vi "18-1.vi"() -> ()   [LabVIEW 2019, in "18.lvlib"]
uses:
  18.lvlib
panel:
  in  "Sample?":bool
  out "Snailfish Number Sum Magnitude":u64
  in  "Sample Index":i32
  out "Snailfish Number Sum Result":string
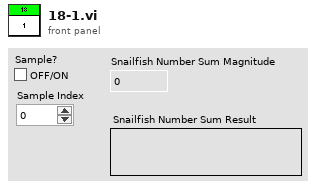
[diagram p1: front panel]
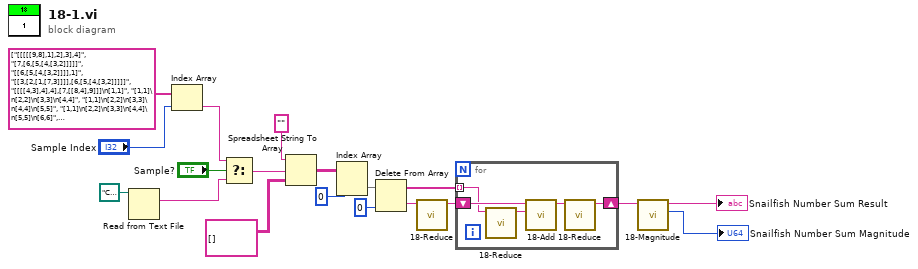
[diagram p0: block diagram]
diagram:
  n1 = Read from Text File(file (use dialog)=path "C:/Users/craig.walker/Documents/GitHub/lv2019-Advent-of-Code-2021/18/input.txt") -> (text=w2:string)  [unwired: 3 in, 3 out]
  n2 = Index Array(array=string[] ["[[[[[9,8],1],2],3],4]", "[7,[6,[5,[4,[3,2]]]]]", "[[6,[5,[4,[3,2]]]],1]", "[[3,[2,[1,[7,3]]]],[6,[5,[4,[3,2]]]]]", "[[[[4,3],4],4],[7,[[8,4],9]]]\n[1,1]", "[1,1]\n[2,2]\n[3,3]\n[4,4]", "[1,1]\n[2,2]\n[3,3]\n[4,4]\n[5,5]", "[1,1]\n[2,2]\n[3,3]\n[4,4]\n[5,5]\n[6,6]", "[[[0,[4,5]],[0,0]],[[[4,5],[2,6]],[9,5]]]\n[7,[[[3,7],[4,3]],[[6,3],[8,8]]]]\n[[2,[[0,8],[3,4]]],[[[6,7],1],[7,[1,6]]]]\n[[[[2,4],7],[6,[0,5]]],[[[6,8],[2,8]],[[2,1],[4,5]]]]\n[7,[5,[[3,8],[1,4]]]]\n[[2,[2,2]],[8,[8,1]]]\n[2,9]\n[1,[[[9,3],9],[[9,0],[0,7]]]]\n[[[5,[7,4]],7],1]\n[[[[4,2],2],6],[8,7]]", "[9,1]", "[[[0,[5,8]],[[1,7],[9,6]]],[[4,[1,2]],[[1,4],2]]]\n[[[5,[2,8]],4],[5,[[9,9],0]]]\n[6,[[[6,2],[5,6]],[[7,6],[4,7]]]]\n[[[6,[0,7]],[0,9]],[4,[9,[9,0]]]]\n[[[7,[6,4]],[3,[1,3]]],[[[5,5],1],9]]\n[[6,[[7,3],[3,2]]],[[[3,8],[5,7]],4]]\n[[[[5,4],[7,7]],8],[[8,3],8]]\n[[9,3],[[9,9],[6,[4,9]]]]\n[[2,[[7,7],7]],[[5,8],[[9,3],[0,2]]]]\n[[[[5,2],5],[8,[3,7]]],[[5,[7,5]],[4,4]]]"], index="Sample Index") -> (element=w3:string)
  n3 = Select(t=w3, s="Sample?", f=w2) -> (s? t:f=w4:string)
  n4 = Spreadsheet String To Array(format string="" ("spreadsheet string"), spreadsheet string=w4, array type (2D Dbl)=string[][] [] ("spreadsheet string")) -> (array=w17:string[][])  [unwired: 1 in]
  n5 = Index Array(array=w17, index (col)=0 ("disabled index (col)")) -> (element=w16:string[])  [unwired: 1 in]
  n6 = Delete From Array(array=w16, index=0) -> (deleted portion=w10:string, array with subset deleted=w15:string[])  [unwired: 1 in]
  n7 = call "18-Reduce.vi"("Snailfish Number in"=w10) -> ("Snailfish Number out"=w9:string)  [unwired: 10 in]
  n8 = for {
    tunnel: w15 -> [w20] mode=indexing
    shift-right: [w22] -> w8
    shift-left: w9 -> [w24]
    n9 = call "18-Reduce.vi"("Snailfish Number in"=w20) -> ("Snailfish Number out"=w21:string)  [unwired: 10 in]
    n10 = call "18-Add.vi"("Snailfish Number y"=w21, "Snailfish Number x"=w24) -> ("Snailfish Number x+y"=w23:string)  [unwired: 9 in]
    n11 = call "18-Reduce.vi"("Snailfish Number in"=w23) -> ("Snailfish Number out"=w22:string)  [unwired: 10 in]
  }
  n12 = call "18-Magnitude.vi"("Snailfish Number in"=w8) -> ("Snailfish Number Magnitude"=→"Snailfish Number Sum Magnitude":u64, "Snailfish Number out"=→"Snailfish Number Sum Result":string)  [unwired: 9 in]
